vi "Get PCL Decimation.vi"(8 "Error In":errorcluster, 11 "Instrument Addon Refnum In":T1 format="%.0x") -> (0 "Error Out":errorcluster, 2 "PCL Decimation":u32, 3 "Instrument Addon Refnum Out":T1=18446744073709551615 format="%.0x")   [LabVIEW 2018, in "Instrument Addon Scripting API.lvlib"]
doc: "Returns the PCL Decimation value set for the Instrument Addon Custom Device\n\nInput:\nInstrument Addon Refnum In: represents the refference number to an Instrument Addon Custom Device\n\nOutput:\nInstrument Addon Refnum Out: represents the refference number to the Instrument Addon Custom Device provided as an input\nPCL Decimation: represents the PCL Decimation Value of the Instrument Addon Custom Device"
uses:
  Instrument Addon Scripting API.lvlib
  <vilib>/NI Veristand/Custom Device API/Custom Device Item Ref.ctl
  Addon/Addon Shared/SubVIs/Constants.vi
  <vilib>/NI/NI VeriStand Advanced SysDef API/_SubVIs/SysDef.Property.Get.U32.vi
  <vilib>/NI/NI VeriStand Advanced SysDef API/SysDef API/Advanced System Definition.lvlib
  Addon/Addon Shared/Instrument Addon Shared.lvlib
  <vilib>/NI Veristand/Custom Device API/Custom Device API.lvlib
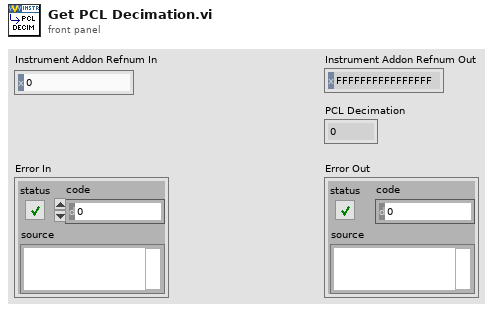
[diagram p1: front panel]
types:
  T1 = typedef "Custom Device API.lvlib/Custom Device Item Ref.ctl" = u64
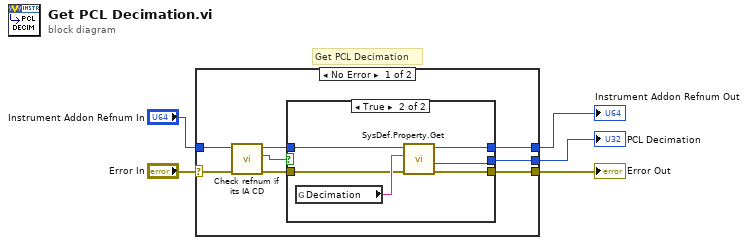
[diagram p0: block diagram]
diagram:
  # "Get PCL Decimation"
  n1 = case shown="No Error" "Error In" {
    selector: "Error In" -> [w13 w23]
    tunnel: "Instrument Addon Refnum In" -> [w11 w22]
    tunnel: [w8 _] -> w4
    tunnel: [w9 w23] -> w3
    tunnel: [w7 w22] -> w1
    frame No Error {
      n2 = call "Check refnum if its IA CD.vi"("Error In"=w13, "Refnum In"=w11) -> ("Error Out"=w12:errorcluster, "Is Instrument Addon?"=w10:bool, "Refnum Out"=w6:u64)  [unwired: 7 in]
      n3 = case shown="True" w10 {
        tunnel: w12 -> [w15 w16]
        tunnel: [w15 w20] -> w9
        tunnel: [_ w19] -> w8
        tunnel: [w14 w18] -> w7
        tunnel: w6 -> [w14 w17]
        frame False {
        }
        frame True {
          n4 = global read "Constants.vi" "Decimation"() -> (w21:string)
          n5 = call-poly <vilib>:"SysDef.Property.Get.vi"("error in (no error)"=w16, "Property Name"=w21, "nodeID"=w17) -> ("error out"=w20:errorcluster, "Value out"=w19:u32, "nodeID out"=w18:u64)  [unwired: 5 in, 1 out]
        }
      }
    }
    frame Error {
    }
  }
  "PCL Decimation" <- w4
  "Error Out" <- w3
  "Instrument Addon Refnum Out" <- w1
